vi "Add Piece Pixels on Board.vi"(8 "error in (no error)":errorcluster caption="entrée d'erreur (pas d'erreur)", 11 "Game Board en entrée":refnum<class "Game Board.lvclass">) -> (0 "error out":errorcluster caption="sortie d'erreur", 3 "Game Board en sortie":refnum<class "Game Board.lvclass">)   [LabVIEW 2017, in "Game Board.lvclass"]
uses:
  Game Board.lvclass
  Game Board.lvclass/Game Board.ctl
  Piece of Bricks_class/Piece of Bricks.lvclass
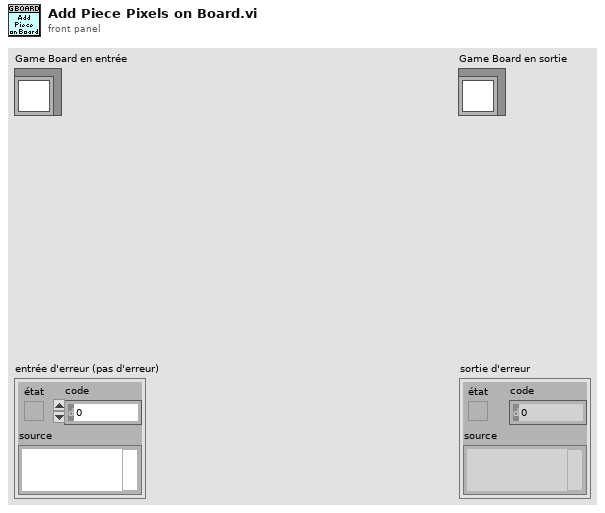
[diagram p1: front panel]
types:
  T1 = typedef "Coordinates.ctl" = cluster{"X":i32, "Y":i32}
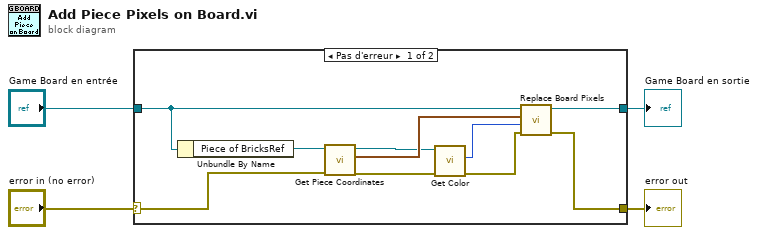
[diagram p0: block diagram]
diagram:
  n1 = case shown="Pas d'erreur" "error in (no error)" {
    selector: "error in (no error)" -> [w7 w16]
    tunnel: [w5 w16] -> w3
    tunnel: [w13 w15] -> w1
    tunnel: "Game Board en entrée" -> [w14 w15]
    frame No Error {
      n2 = Unbundle By Name(w14) -> ("Piece of BricksRef"=w12:refnum<class "Piece of Bricks.lvclass">)
      n3 = call-dynamic "Get Piece Coordinates.vi"("error in (no error)"=w7, "object in"=w12) -> ("error out"=w8:errorcluster, "Piece Coordinates"=w11:T1[], "object out"=w10:refnum<class "Piece of Bricks.lvclass">)  [unwired: 7 in]
      n4 = call-dynamic "Get Color.vi"("error in (no error)"=w8, "object in"=w10) -> ("error out"=w6:errorcluster, "Color"=w9:u32)  [unwired: 7 in, 1 out]
      n5 = call-dynamic "Replace Board Pixels.vi"("error in (no error)"=w6, "New pixels color"=w9, "Pixels"=w11, "Game Board en entrée"=w14) -> ("error out"=w5:errorcluster, "Game Board en sortie"=w13:refnum<class "Game Board.lvclass">)  [unwired: 6 in]
    }
    frame Error {
    }
  }
  "error out" <- w3
  "Game Board en sortie" <- w1
